vi "IsError.vi"(11 "error in (no error)":errorcluster) -> (3 "Boolean":bool)   [LabVIEW 2019]
panel:
  # "This really isn't needed ...."
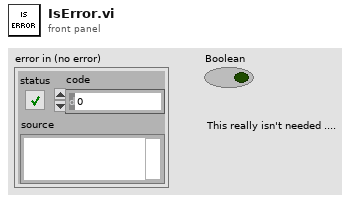
[diagram p1: front panel]
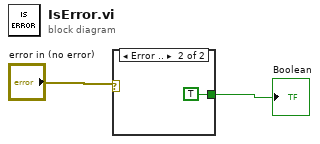
[diagram p0: block diagram]
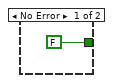
[diagram p2: hidden frame]
diagram:
  n1 = case shown="Error .." "error in (no error)" {
    tunnel: [FALSE TRUE] -> w2
    frame No Error {
    }
    frame Error {
    }
  }
  "Boolean" <- w2
